vi "currentLocation.vi"(11 "Equip_Data":T1 {"integration_time_dataSet"."dset_ref" format="%.0x"; "instrument_dataSet"."dset_ref" format="%.0x"; "h5File_refOut" format="%.0x"}) -> (0 "error out":errorcluster, 3 "position":cluster{"X":dbl, "Y":dbl, "Z":dbl})   [LabVIEW 2015]
uses:
  controls/Equip_Data.ctl
  <vilib>/Utility/miscctls.llb/LV3DPointTypeDef.ctl
  controls/startScanData.ctl
  controls/scanInstrumentInfo.ctl
  <vilib>/addons/h5labview2/base/hid_t.ctl
  controls/HDF5_Dset_4d.ctl
  controls/HDF5_Dset_3d.ctl
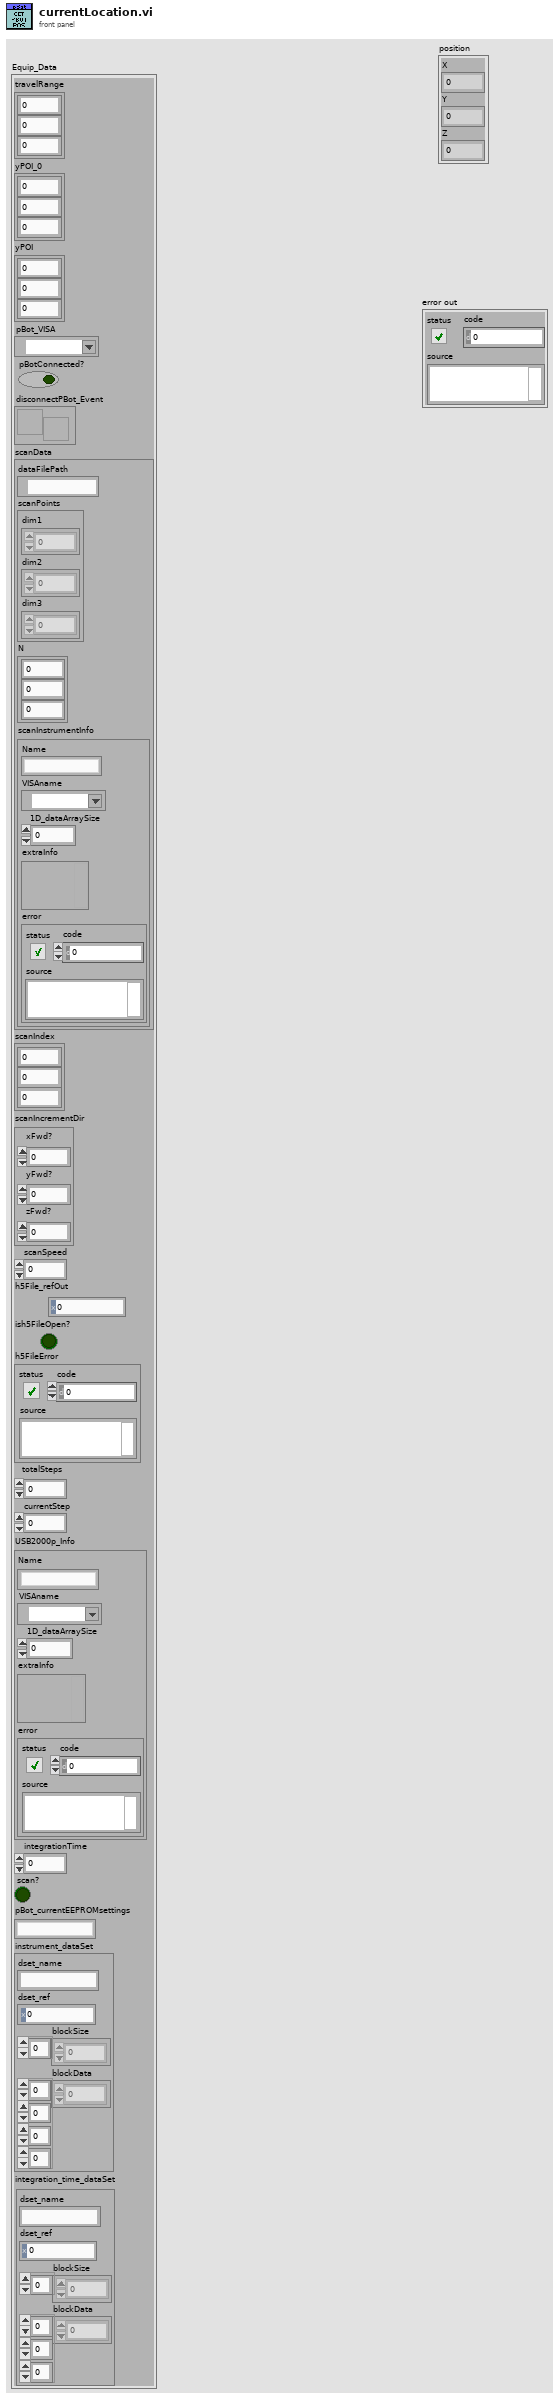
[diagram p1: front panel]
types:
  T1 = typedef "Equip_Data.ctl" = cluster{"travelRange":T2, "yPOI_0":T2, "yPOI":T2, "pBot_VISA":refnum<visa-resource-name>, "pBotConnected?":bool, "disconnectPBot_Event":refnum<user-event>, "scanData":T3, "scanIndex":cluster{"X":u16, "Y":u16, "Z":u16}, "scanIncrementDir":cluster{"xFwd?":i16, "yFwd?":i16, "zFwd?":i16}, "scanSpeed":u16, "h5File_refOut":T5, "ish5FileOpen?":bool, "h5FileError":errorcluster, "totalSteps":u32, "currentStep":u32, "USB2000p_Info":T4, "integrationTime":u32, "scan?":bool, "pBot_currentEEPROMsettings":string, "instrument_dataSet":T6, "integration_time_dataSet":T7}
  T2 = typedef "LV3DPointTypeDef.ctl" = cluster{"X":sgl, "Y":sgl, "Z":sgl}
  T3 = typedef "startScanData.ctl" = cluster{"dataFilePath":path, "scanPoints":cluster{"dim1":sgl[], "dim2":sgl[], "dim3":sgl[]}, "N":cluster{"X":u16, "Y":u16, "Z":u16}, "scanInstrumentInfo":T4}
  T4 = typedef "scanInstrumentInfo.ctl" = cluster{"Name":string, "VISAname":refnum<visa-resource-name>, "1D_dataArraySize":u16, "extraInfo":variant, "error":errorcluster}
  T5 = typedef "hid_t.ctl" = i32
  T6 = typedef "HDF5_Dset_4d.ctl" = cluster{"dset_name":string, "dset_ref":T5, "blockSize":u16[], "blockData":u16[][][][]}
  T7 = typedef "HDF5_Dset_3d.ctl" = cluster{"dset_name":string, "dset_ref":T5, "blockSize":u16[], "blockData":u32[][][]}
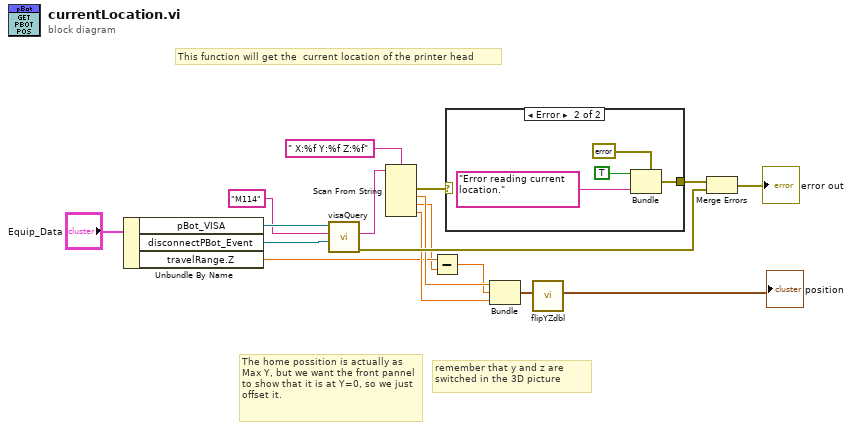
[diagram p0: block diagram]
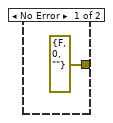
[diagram p2: hidden frame]
diagram:
  # "The home possition is actually as Max Y, but we want the front pannel to show that it is at Y=0, so we just offset it."
  # "remember that y and z are switched in the 3D picture"
  # "This function will get the  current location of the printer head"
  n1 = Unbundle By Name("Equip_Data") -> ("pBot_VISA"=w8:refnum<visa-resource-name>, "disconnectPBot_Event"=w7:refnum<user-event>, "travelRange.Z"=w5:sgl)
  n2 = call "visaQuery.vi"("disconnectPBot_Event"=w7, "stringToWrite"="M114" ("format string"), "VISA resource name"=w8) -> ("error Out"=w16:errorcluster, "String"=w13:string)  [unwired: 6 in, 1 out]
  n3 = Scan From String(format string=" X:%f Y:%f Z:%f", input string=w13) -> (error out=w14:errorcluster, output 1=w11:dbl, output 2=w4:dbl, output 3=w10:dbl)  [unwired: 5 in, 2 out]
  n4 = Subtract(x=w5, y=w4) -> (x-y=w3:dbl)
  n5 = case shown="Error" w14 {
    tunnel: [errorcluster {"status"=FALSE, "code"=0, "source"=""} ("error constant") w20] -> w15
    frame No Error {
    }
    frame Error {
      n6 = Bundle(cluster=errorcluster {"status"=TRUE, "code"=0, "source"=""} ("error constant"), "status"=TRUE, "source"="Error reading current location." ("format string")) -> (w20:errorcluster)  [unwired: 1 in]
    }
  }
  n7 = Bundle(w11, w3, w10) -> (w9:cluster{dbl, dbl, dbl})  [unwired: 1 in]
  n8 = call "flipYZdbl.vi"("pointIn"=w9) -> ("pointOut"=→"position":cluster{"X":dbl, "Y":dbl, "Z":dbl})  [unwired: 10 in]
  n9 = Merge Errors(w15, w16) -> (→"error out":errorcluster)
